vi "DryerReadWrite.vi"(0 "Com Chan":u8, 7 "Dryer Status Serial Data In":T1, 11 "error in (no error)":errorcluster) -> (4 "Dryer Status Serial Data":T1, 6 "Read Buffer":string, 8 "Log String":string, 15 "error out":errorcluster)   [LabVIEW 2012]
uses:
  Dryer Com Port Info.ctl
  Dryer Status Ctrl.ctl
  GEA2 Driver/GEA2 Dryer Interface Ctrl.ctl
  Globals Wilt.vi
panel:
  out "x-y 3":u32
  out "x-y 2":u32
  out "x-y":u32
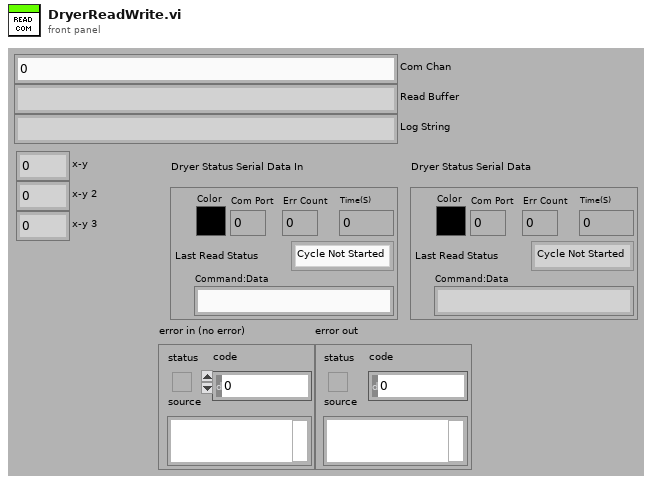
[diagram p1: front panel]
types:
  T1 = typedef "Dryer Com Port Info.ctl" = cluster{"Color":u32, "Last Read Status":T2, "Command:Data":string, "Com Port":u8, "Time(S)":dbl, "Err Count":u32}
  T2 = typedef "Dryer Status Ctrl.ctl" = enum16{"Cycle Not Started", "Cycle Running", "Paused", "Cycle Completed", "Eval Mode Entered", "Err", "Pause (No GEA2)"}
  T3 = typedef "GEA2 Dryer Interface Ctrl.ctl" = enum16{"Init Com Port", "SendCMD", "ReadPort", "Close Port", "Simulate Diag Data", "Simulate Dryer", "Send WILT Startup CMDs", "Send Continue CMD", "Read Continuous"}
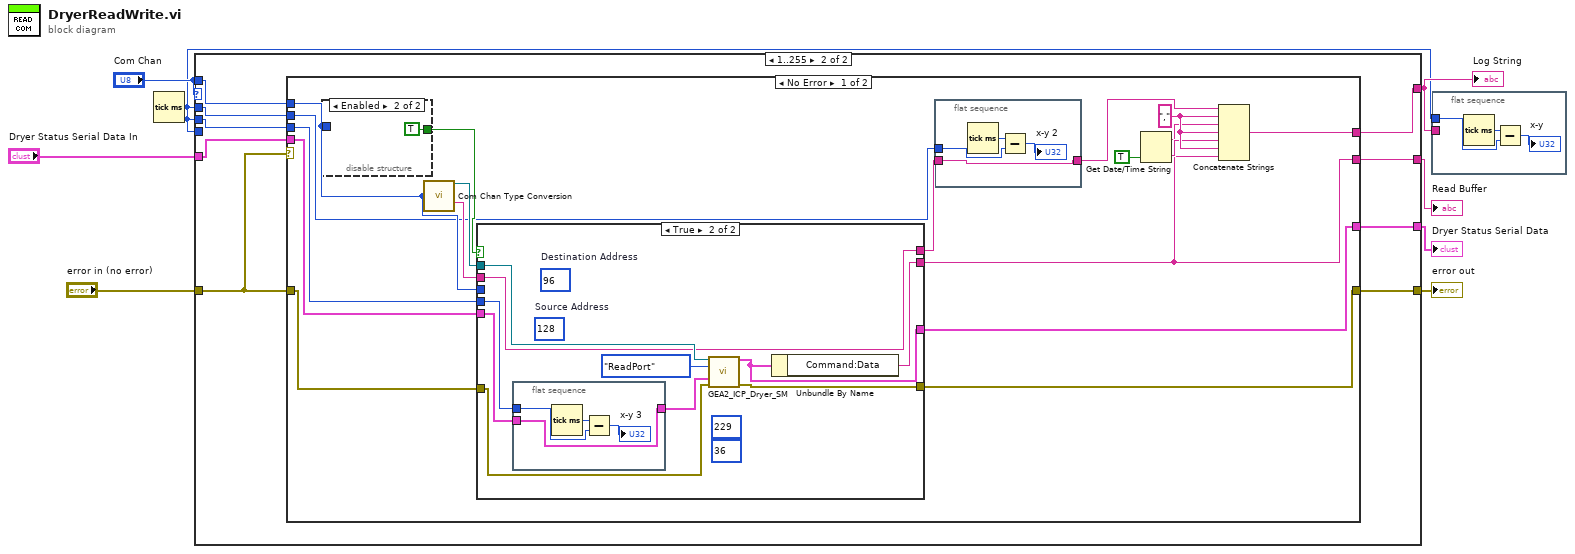
[diagram p0: block diagram]
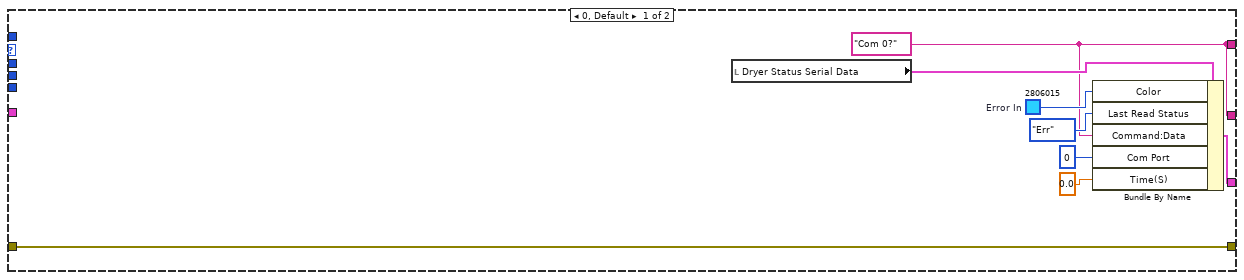
[diagram p2: hidden frame]
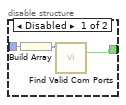
[diagram p3: hidden frame]
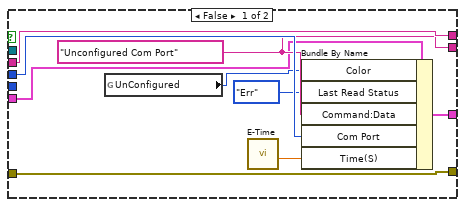
[diagram p4: hidden frame]
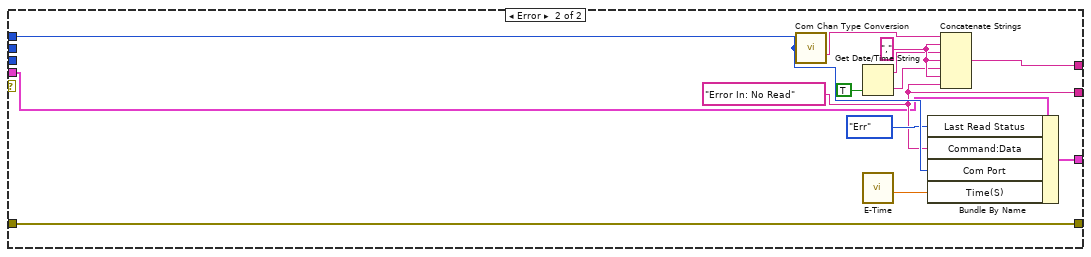
[diagram p5: hidden frame]
diagram:
  n1 = Tick Count (ms)() -> (millisecond timer value=w1:u32)
  n2 = case shown="1..255" "Com Chan" {
    tunnel: "Com Chan" -> [_ w25]
    tunnel: [w16 w24] -> w8
    tunnel: "error in (no error)" -> [w16 w23]
    tunnel: [w12 w22] -> w2
    tunnel: [w12 w21] -> w5
    tunnel: [w9 w20] -> w4
    tunnel: "Dryer Status Serial Data In" -> [_ w19]
    tunnel: w1 -> [_ _]
    tunnel: w1 -> [_ w18]
    tunnel: w1 -> [_ w17]
    frame 0, Default {
      w13 = u32 2806015  # Error In
      w12 = "Com 0?" ("ASCII Data")
      n3 = local read "Dryer Status Serial Data"() -> (w15:T1)
      n4 = Bundle By Name(cluster=w15, "Color"=w13, "Last Read Status"=Dryer_Status_Ctrl."Err" ("Status"), "Command:Data"=w12, "Com Port"=u8 0, "Time(S)"=0.0) -> (w9:T1)
    }
    frame 1..255 {
      n5 = case shown="No Error" w23 {
        tunnel: w25 -> [w34 w81]
        tunnel: [w43 w87] -> w24
        tunnel: w23 -> [w42 w87]
        tunnel: [w33 w78] -> w22
        tunnel: [w32 w77] -> w21
        tunnel: [w31 w76] -> w20
        tunnel: w19 -> [w30 w75]
        tunnel: w18 -> [w27 _]
        tunnel: w17 -> [w26 _]
        frame No Error {
          w38 = "," ("string")
          n6 = disable-structure shown="Enabled" {
            disable-tunnel: [w45 TRUE ("Found?")] -> w39
            disable-tunnel: w34 -> [w44 _]
            frame Disabled {
              n7 = Build Array(w44) -> (w46:u8[])
              n8 = call "Find Valid Com Ports.vi"("Valid Com Port List(100,2:56)"=w46) -> ("Found?"=w45:bool)  [unwired: 13 in, 1 out]
            }
            frame Enabled {
            }
          }
          n9 = call "Com Chan Type Conversion.vi"("Com Chan"=w34) -> ("VISA resource name"=w41:refnum<visa-resource-name>, "Com Text"=w40:string)  [unwired: 11 in, 2 out]
          n10 = case shown="True" w39 {
            tunnel: [w55 w70] -> w43
            tunnel: w42 -> [w55 w69]
            tunnel: w41 -> [_ w68]
            tunnel: w40 -> [w60 w64]
            tunnel: [w59 w66] -> w31
            tunnel: [w57 w65] -> w32
            tunnel: [w60 w64] -> w28
            tunnel: w34 -> [w58 _]
            tunnel: w30 -> [w53 w63]
            tunnel: w26 -> [_ w61]
            frame False {
              w57 = "Unconfigured Com Port" ("ASCII Data")
              n11 = global read "Globals Wilt.vi" "UnConfigured"() -> (w52:u32)
              n12 = call "E-Time.vi"() -> ("Elapsed Time (sec)"=w54:dbl)  [unwired: 9 in, 2 out]
              n13 = Bundle By Name(cluster=w53, "Color"=w52, "Last Read Status"=Dryer_Status_Ctrl."Err" ("Status"), "Command:Data"=w57, "Com Port"=w58, "Time(S)"=w54) -> (w59:T1)
            }
            frame True {
              (unwired) u8 36 ("Destination Address")
              (unwired) u8 229 ("Source Address")
              (unwired) u8 128  # Source Address
              (unwired) u8 96  # Destination Address
              n14 = flat-sequence {
                tunnel: [w74] -> w62
                tunnel: w63 -> [w74]
                tunnel: w61 -> [w72]
                frame #0 {
                  n15 = Tick Count (ms)() -> (millisecond timer value=w73:u32)
                  n16 = Subtract(x=w73, y=w72) -> (x-y=→"x-y 3":u32)
                }
              }
              n17 = call "GEA2_ICP_Dryer_SM.vi"("ComPort"=w68, "Mode"=GEA2_Dryer_Interface_Ctrl."ReadPort", "Dryer Status Serial Data In"=w62, "Error In"=w69) -> ("Dryer Status Serial Data Out"=w66:T1, "Error Out"=w70:errorcluster)  [unwired: 6 in, 4 out]
              n18 = Unbundle By Name(w66) -> ("Command:Data"=w65:string)
            }
          }
          n19 = flat-sequence {
            tunnel: [w51] -> w29
            tunnel: w28 -> [w51]
            tunnel: w27 -> [w49]
            frame #0 {
              n20 = Tick Count (ms)() -> (millisecond timer value=w50:u32)
              n21 = Subtract(x=w50, y=w49) -> (x-y=→"x-y 2":u32)
            }
          }
          n22 = Get Date/Time String(want seconds? (F)=TRUE) -> (date string=w36:string, time string=w37:string)  [unwired: 2 in]
          n23 = Concatenate Strings(w29, w38, w36, w38, w37, w38, w32) -> (w33:string)
        }
        frame Error {
          w77 = "Error In: No Read" ("ASCII Data")
          w86 = "," ("string")
          n24 = call "Com Chan Type Conversion.vi"("Com Chan"=w81) -> ("Com Text"=w82:string)  [unwired: 11 in, 3 out]
          n25 = Get Date/Time String(want seconds? (F)=TRUE) -> (date string=w84:string, time string=w85:string)  [unwired: 2 in]
          n26 = call "E-Time.vi"() -> ("Elapsed Time (sec)"=w79:dbl)  [unwired: 9 in, 2 out]
          n27 = Bundle By Name(cluster=w75, "Last Read Status"=Dryer_Status_Ctrl."Err" ("Status"), "Command:Data"=w77, "Com Port"=w81, "Time(S)"=w79) -> (w76:T1)
          n28 = Concatenate Strings(w82, w86, w84, w86, w85, w86, w77) -> (w78:string)
        }
      }
    }
  }
  "error out" <- w8
  "Log String" <- w2
  "Read Buffer" <- w5
  "Dryer Status Serial Data" <- w4
  n29 = flat-sequence {
    tunnel: w2 -> [_]
    tunnel: w1 -> [w89]
    frame #0 {
      n30 = Tick Count (ms)() -> (millisecond timer value=w90:u32)
      n31 = Subtract(x=w90, y=w89) -> (x-y=→"x-y":u32)
    }
  }
